vi "rOUTING_sCRIPT.vi"(5 "Part?":bool, 7 "Table":string, 8 "error in (no error)":errorcluster, 11 "Data":T1[](array[typedef])) -> (0 "error out":errorcluster, 3 "spreadsheet string":string)   [LabVIEW 2020]
uses:
  Controls/Routing.ctl
  <menus>/Controls/Devaseelan Style/ONOFF Small.ctl
  <userlib>/_OpenG.lib/array/array.llb/Search 1D Array (String)__ogtk.vi
  MS SQL/MS_Global.vi
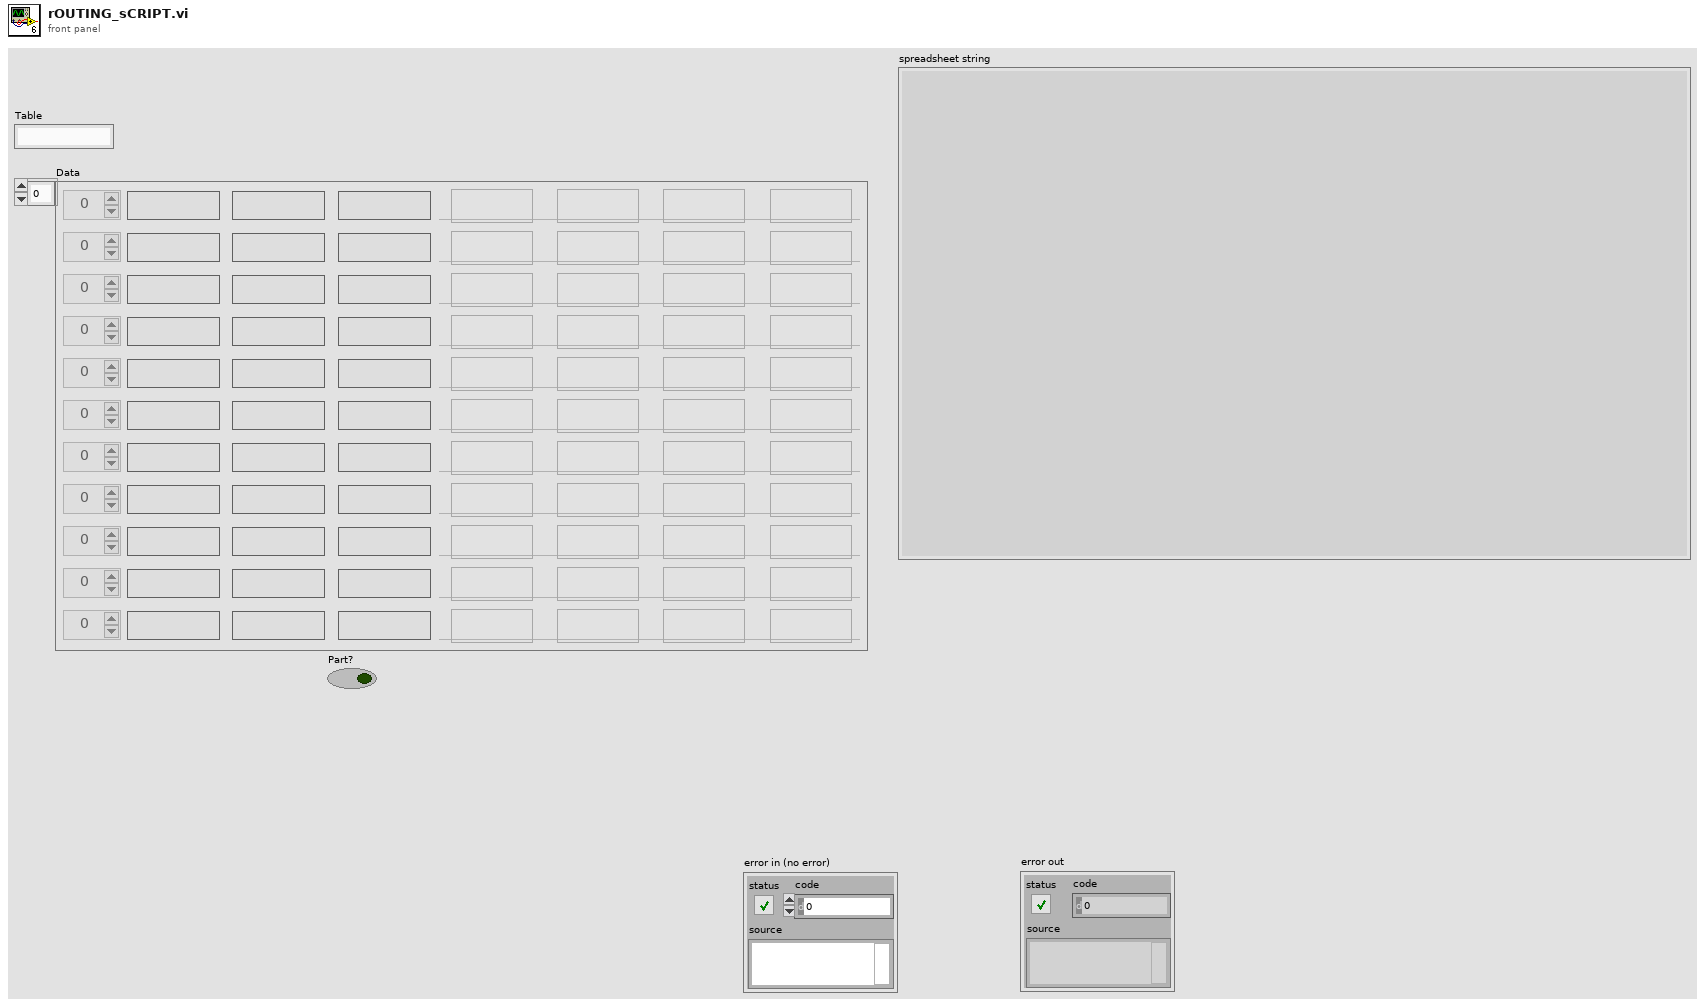
[diagram p1: front panel]
types:
  T1 = typedef "Routing.ctl" = cluster{"OperationSeqNo":i32, "Table Code":string, "OperationCode":string, "MachineCode":string, "OperationRequired":T2, "Traceability":T2, "POKA_YOKE_ALLOWED":T2, "Engraving":T2}
  T2 = typedef "ONOFF Small.ctl" = bool
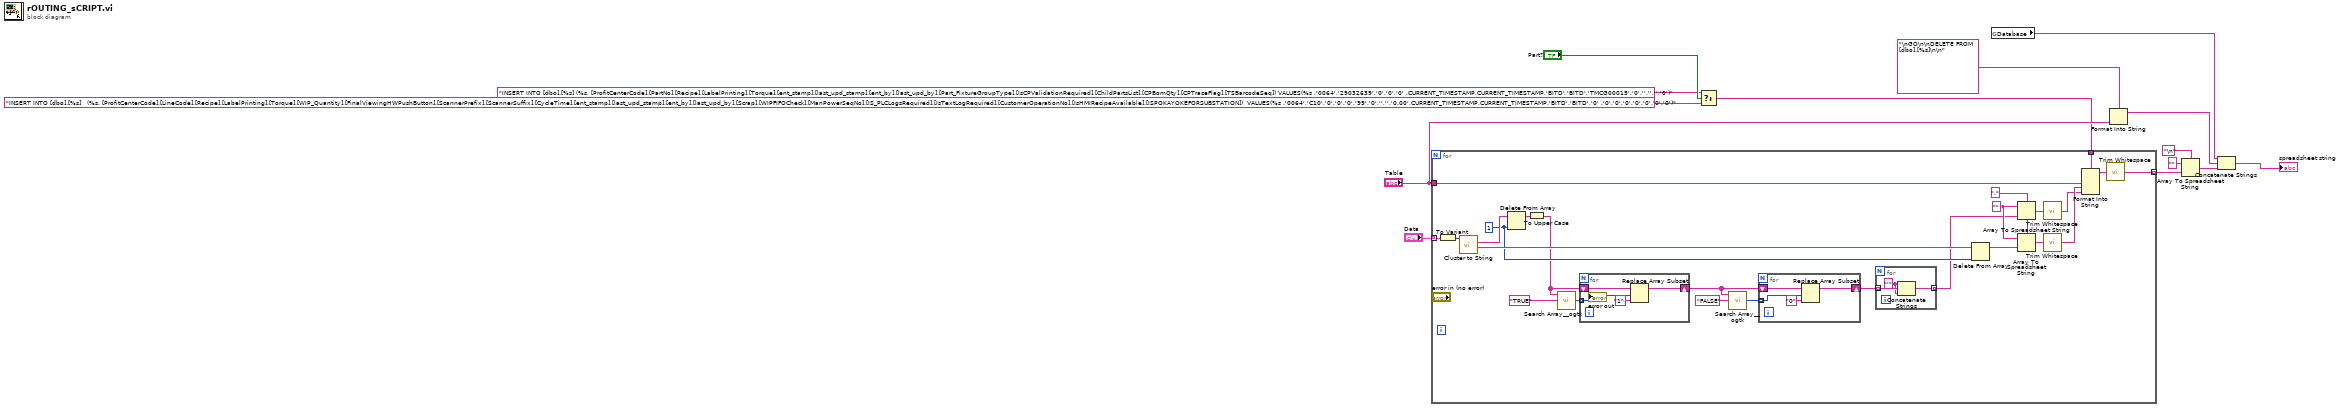
[diagram p0: block diagram]
diagram:
  n1 = Select(t="INSERT INTO [dbo].[%s] (%s, [ProfitCenterCode],[PartNo],[Recipe],[LabelPrinting],[Torque],[ent_stamp],[last_upd_stamp],[ent_by],[last_upd_by],[Part_FixtureGroupType],[IsCPValidationRequired],[ChildPartsList],[CPBomQty],[CPTraceFlag],[TSBarcodeSeq]) VALUES(%s ,'0064','29032639','0','0','0' ,CURRENT_TIMESTAMP,CURRENT_TIMESTAMP,'BITD','BITD','TMCG00015','0','','','','0')" ("delimiter (Tab)"), s="Part?", f="INSERT INTO [dbo].[%s]   (%s, [ProfitCenterCode],[LineCode],[Recipe],[LabelPrinting],[Torque],[WIP_Quantity],[FinalViewingHWPushButton],[ScannerPrefix],[ScannerSuffix],[CycleTime],[ent_stamp],[last_upd_stamp],[ent_by],[last_upd_by],[Scrap],[WIPFIFOCheck],[ManPowerSeqNo],[IS_PLCLogsRequired],[IsTextLogRequired],[CustomerOperationNo],[IsHMIRecipeAvailable],[ISPOKAYOKEFORSUBSTATION])  VALUES(%s ,'0064','C10','0','0','0','99','0','','','0.00',CURRENT_TIMESTAMP,CURRENT_TIMESTAMP,'BITD','BITD','0' ,'0','0','0','0','0','0','0')" ("delimiter (Tab)")) -> (s? t:f=w1:string)
  n2 = for {
    tunnel: "Data" -> [w39] mode=indexing
    tunnel: w1 -> [w31]
    tunnel: "Table" -> [w30]
    tunnel: [w26] -> w11 mode=indexing
    w32 = "," ("delimiter (Tab)")
    w33 = "" ("format string")
    w35 = 1 ("index")
    n3 = To Variant(anything=w39) -> (Variant=w38:variant)
    n4 = call <userlib>:"Cluster to String.vi"("Variant In"=w38) -> ("Format String Name"=w36:string[], "Format String Array"=w37:string[])  [unwired: 7 in, 2 out]
    n5 = Delete From Array(array=w37, index=w35) -> (array with subset deleted=w17:string[])  [unwired: 1 in, 1 out]
    n6 = To Upper Case(1:w17) -> (0:w18:string[])
    n7 = call-poly <userlib>:"Search Array__ogtk.vi"("Array"=w18, "Element Data"="TRUE") -> ("Indices of Elements"=w22:i32[])  [unwired: 7 in]
    n8 = for {
      tunnel: w22 -> [w46] mode=indexing
      shift-right: [w44] -> w19
      shift-left: w18 -> [w47]
      n9 = Replace Array Subset(array=w47, new element="1" ("new element/subarray"), index=w46) -> (w44:string[])
    }
    n10 = call-poly <userlib>:"Search Array__ogtk.vi"("Array"=w19, "Element Data"="FALSE") -> ("Indices of Elements"=w21:i32[])  [unwired: 7 in]
    n11 = for {
      tunnel: w21 -> [w42] mode=indexing
      shift-right: [w40] -> w16
      shift-left: w19 -> [w43]
      n12 = Replace Array Subset(array=w43, new element="0" ("new element/subarray"), index=w42) -> (w40:string[])
    }
    n13 = for {
      tunnel: [w49] -> w15 mode=indexing
      tunnel: w16 -> [w50] mode=indexing
      w48 = "'" ("string")
      n14 = Concatenate Strings(w48, w50, w48) -> (w49:string)
    }
    n15 = Delete From Array(array=w36, index=w35) -> (array with subset deleted=w34:string[])  [unwired: 1 in, 1 out]
    n16 = Array To Spreadsheet String(delimiter (Tab)=w32, array=w15, 3:w33) -> (spreadsheet string=w29:string)
    n17 = Array To Spreadsheet String(delimiter (Tab)=w32, array=w34, 3:w33) -> (spreadsheet string=w28:string)
    n18 = call <vilib>:"Trim Whitespace.vi"("string"=w29) -> ("trimmed string"=w24:string)  [unwired: 1 in]
    n19 = call <vilib>:"Trim Whitespace.vi"("string"=w28) -> ("trimmed string"=w25:string)  [unwired: 1 in]
    n20 = Format Into String(format string=w31, w30, w25, w24) -> (resulting string=w27:string)  [unwired: 2 in, 1 out]
    n21 = call <vilib>:"Trim Whitespace.vi"("string"=w27) -> ("trimmed string"=w26:string)  [unwired: 1 in]
  }
  n22 = global read "MS_Global.vi" "Database"() -> (w6:string)
  n23 = Format Into String(format string="\nGO\n\nDELETE FROM [dbo].[%s]\n\n" ("delimiter (Tab)"), "Table") -> (resulting string=w5:string)  [unwired: 2 in, 1 out]
  n24 = Array To Spreadsheet String(delimiter (Tab)="\n", array=w11, 3:"" ("format string")) -> (spreadsheet string=w14:string)
  n25 = Concatenate Strings(w6, w5, w14) -> (→"spreadsheet string":string)
